vi "SignalGenerator+Normalization.vi"() -> ()   [LabVIEW 2021]
uses:
  <vilib>/numeric/Random Number (Range) I64.vi
  <vilib>/numeric/sub_Random U32.vi
panel:
  out "Waveform Chart":waveform(i32)(graph)
  out "output waveform":waveform(i32)
  out "Numeric":i32
  in  "stop":bool
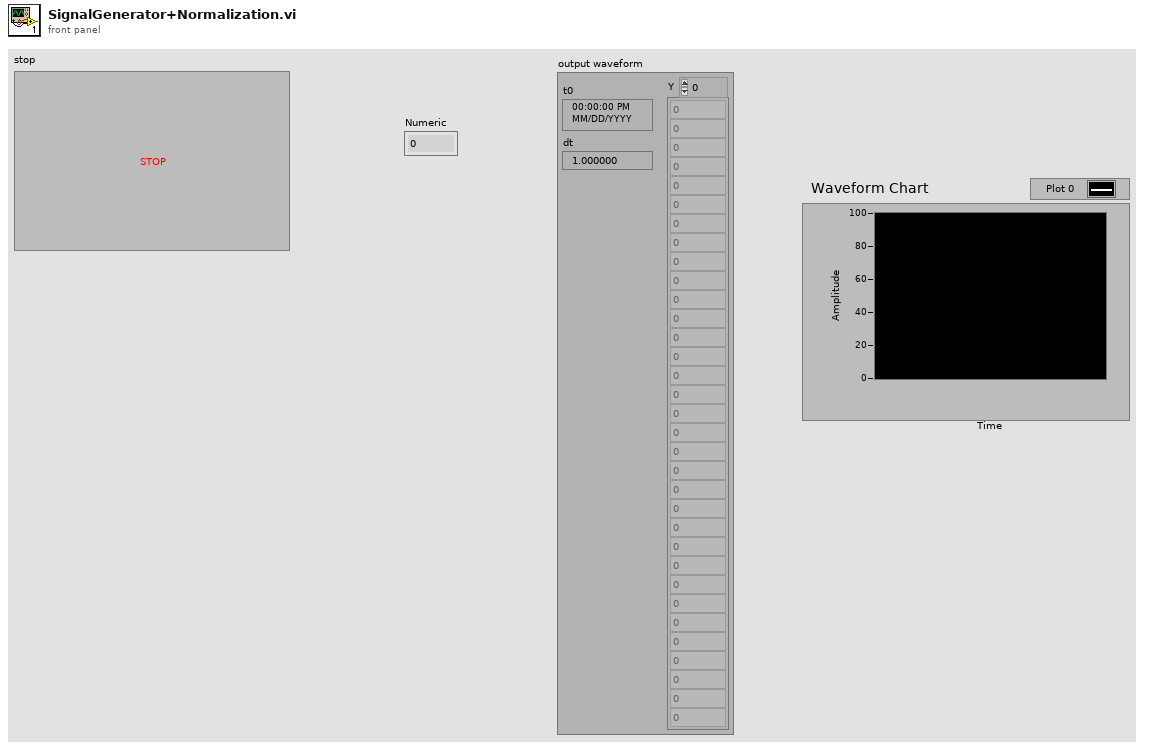
[diagram p1: front panel]
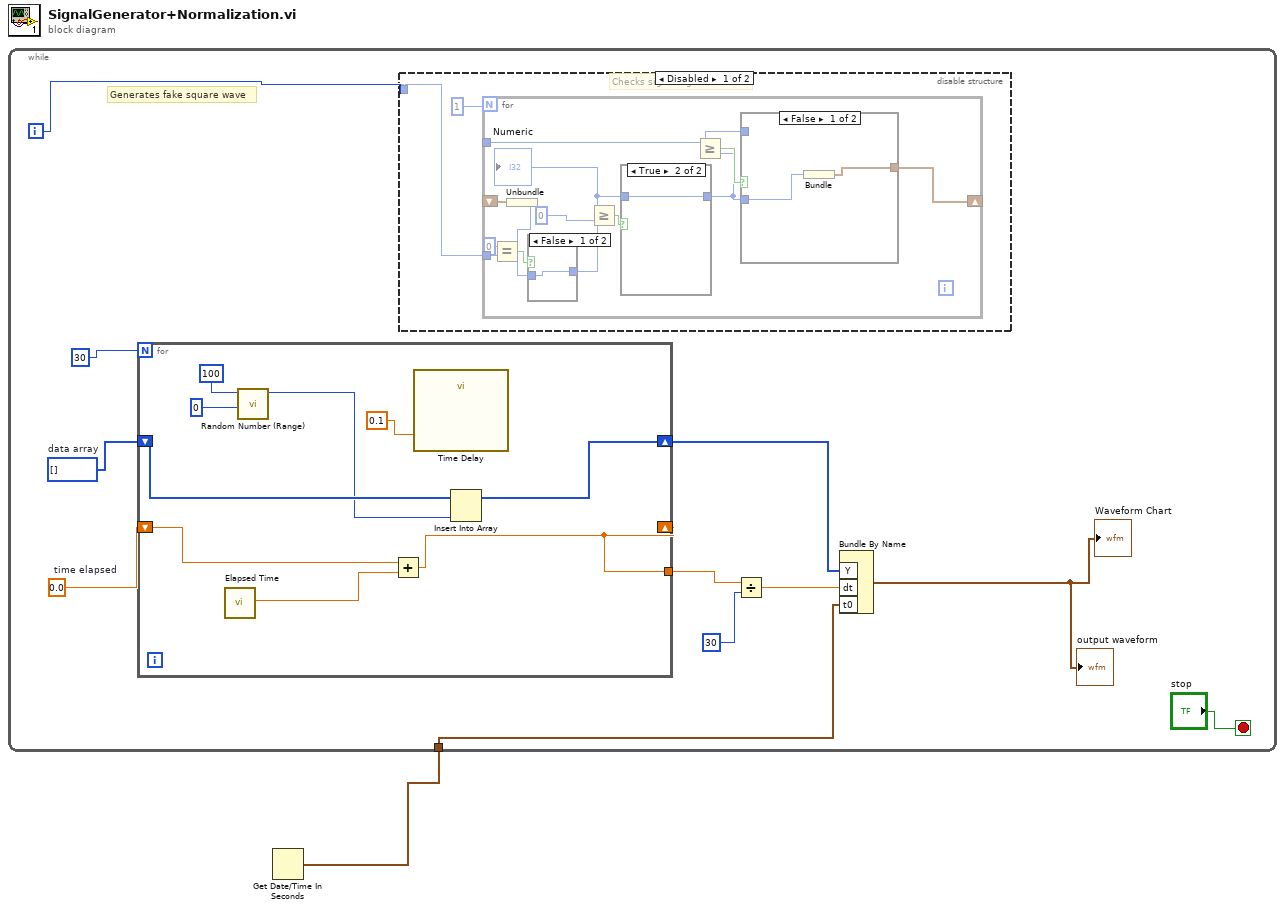
[diagram p0: block diagram]
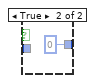
[diagram p2: hidden frame]
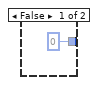
[diagram p3: hidden frame]
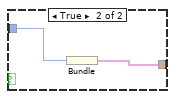
[diagram p4: hidden frame]
diagram:
  n1 = Get Date/Time In Seconds() -> (seconds since 1Jan1904=w1:timestamp)
  n2 = while {
    tunnel: w1 -> [w7]
    i -> [w11]
    stop <- "stop" stop-if-true
    w10 = i32[] []  # data array
    w9 = 0.0  # time elapsed
    # "Generates fake square wave"
    n3 = for {
      N: 30 -> [_]
      shift-right: [w41] -> w8
      shift-left: w10 -> [w42]
      shift-right: [w38] -> _
      shift-left: w9 -> [w40]
      tunnel: [w38] -> w4
      n4 = call "Elapsed Time"() -> ("Elapsed Time (s)"=w43:dbl)  [unwired: 12 in, 7 out]
      n5 = call-poly <vilib>:"Random Number (Range).vi"("lower bound (-100)"=i64 0, "upper bound (100)"=i64 100) -> ("number"=w35:i64)  [unwired: 9 in]
      n6 = Add(x=w40, y=w43) -> (x+y=w38:dbl)
      n7 = call "Time Delay"("Delay Time (s)"=0.1) -> ()  [unwired: 10 in, 1 out]
      n8 = Insert Into Array(array=w42, new element=w35) -> (w41:i32[])  [unwired: 1 in]
    }
    n9 = disable-structure shown="Disabled" {
      disable-tunnel: w11 -> [w13 _]
      frame Disabled {
        # "Checks signal against max"
        n10 = for {
          N: 1 -> [_]
          tunnel: _ -> [w25]
          shift-right: [w24] -> _
          shift-left: _ -> [w23]
          tunnel: w13 -> [w20]
          n11 = Equal?(x=0, y=w20) -> (x = y?=w17:bool)
          n12 = Unbundle(w23) -> (w16:i32)
          n13 = case shown="False" w17 {
            tunnel: w16 -> [w27 _]
            tunnel: [w27 0] -> w15
            frame False {
            }
            frame True {
            }
          }
          "Numeric" <- w15
          n14 = Greater Or Equal?(x=w15, y=0) -> (x >= y?=w22:bool)
          n15 = case shown="True" w22 {
            tunnel: w15 -> [_ w30]
            tunnel: [0 w30] -> w21
            frame False {
            }
            frame True {
            }
          }
          n16 = Greater Or Equal?(x=w25, y=w21) -> (x >= y?=w26:bool)
          n17 = case shown="False" w26 {
            tunnel: w25 -> [_ w34]
            tunnel: [w31 w33] -> w24
            tunnel: w21 -> [w32 _]
            frame False {
              n18 = Bundle(w32) -> (w31:cluster{i32})  [unwired: 1 in]
            }
            frame True {
              n19 = Bundle(w34) -> (w33:cluster{void})  [unwired: 1 in]
            }
          }
        }
      }
      frame Enabled {
      }
    }
    n20 = Divide(x=w4, y=30) -> (x/y=w2:dbl)
    n21 = Bundle By Name("Y"=w8, "dt"=w2, "t0"=w7) -> (→"Waveform Chart" →"output waveform":waveform(i32))  [unwired: 1 in]
  }
